vi "PidHmiFrequencyToInterval.vi"(10 "Frequence":dbl, 11 "Default":i32) -> (3 "Numeric":i32)   [LabVIEW 2018, in "Pid.lvlib"]
uses:
  Pid.lvlib
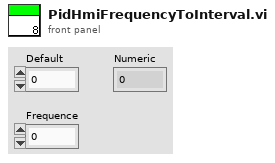
[diagram p1: front panel]
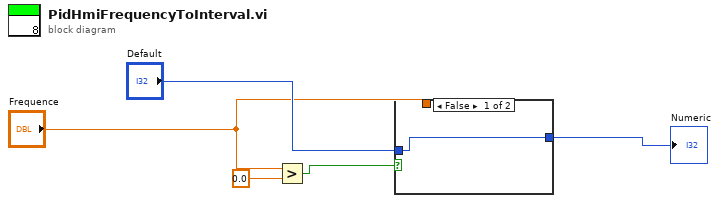
[diagram p0: block diagram]
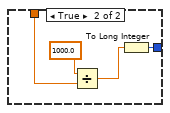
[diagram p2: hidden frame]
diagram:
  n1 = Greater?(x="Frequence", y=0.0) -> (0:w2:bool)
  n2 = case shown="False" w2 {
    tunnel: "Frequence" -> [_ w10]
    tunnel: "Default" -> [w6 _]
    tunnel: [w6 w7] -> w5
    frame False {
    }
    frame True {
      n3 = Divide(x=1000.0, y=w10) -> (x/y=w8:dbl)
      n4 = To Long Integer(number=w8) -> (32bit integer=w7:i32)
    }
  }
  "Numeric" <- w5
